vi "Format String Insert Into.vi"() -> ()   [LabVIEW 2024]
uses:
  <vilib>/addons/database/Connection.llb/Conn ObjectReference.ctl
  <vilib>/addons/database/NI_Database_API.lvlib
panel:
  out "resulting string":string
  in  "Foto":path
  in  "Email":string
  in  "Alamat":string
  in  "Nama":string
  in  "NIM":string
  in  "Boolean":bool
  out "error out":errorcluster
  in  "error in (no error)":errorcluster
  out "connection reference 2":T1
  in  "connection reference":T1
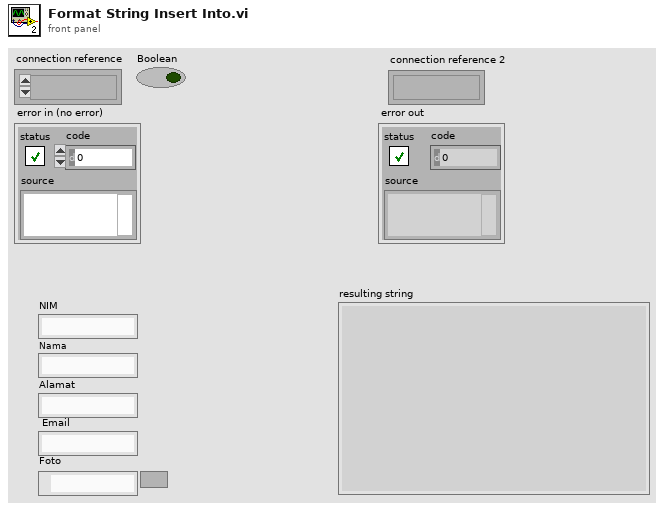
[diagram p1: front panel]
types:
  T1 = typedef "NI_Database_API.lvlib/Conn ObjectReference.ctl" = refnum<k1>
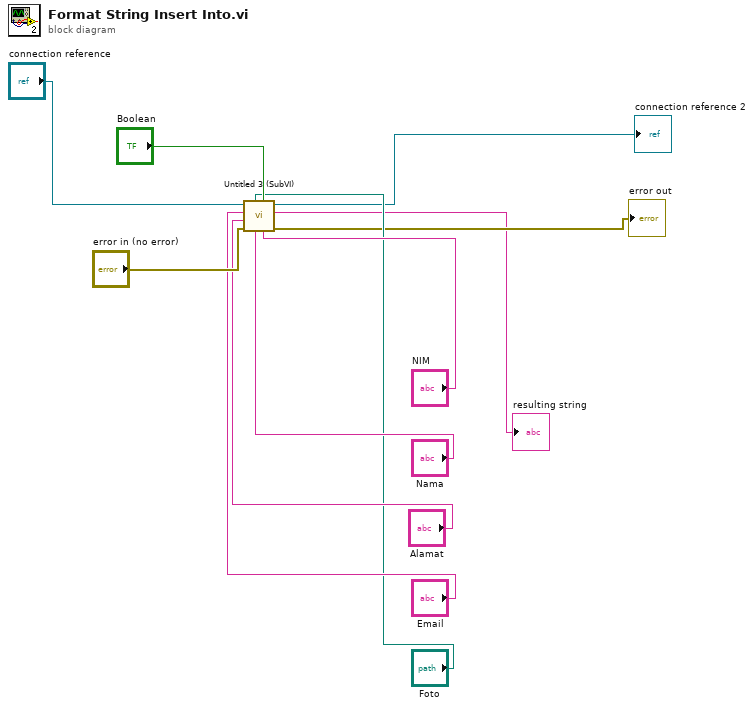
[diagram p0: block diagram]
diagram:
  n1 = call "Untitled 3 (SubVI).vi"("NIM"="NIM", "Boolean"="Boolean", "Nama"="Nama", "Foto"="Foto", "error in (no error)"="error in (no error)", "Alamat"="Alamat", "Email"="Email", "Refnum in"="connection reference") -> ("error out"=→"error out":errorcluster, "resulting string"=→"resulting string":string, "Refnum out"=→"connection reference 2":T1)  [unwired: 1 in]
